vi "Gran result.vi"(6 "first i":u8, 7 "F1":dbl[](array[numeric]) format="%.7f", 8 "length":u8, 9 "Vo":dbl=100.0 format="%.2f", 10 "Nt":dbl=0.05 format="%.2f", 11 "Vt":dbl[](array[numeric]) format="%.5f") -> (0 "graph":cluster{"Vt":dbl[], "F1":dbl[]}[](array[cluster]) {"F1" format="%.2f"; "Vt" format="%.2f"}, 1 "r":dbl=0.5 format="%.6f", 2 "Est. Nt":dbl=0.05 format="%.6f", 3 "ANC":dbl=0.5 format="%.6f", 5 "Ve":dbl=0.5 format="%.6f")   [LabVIEW 2012]
uses:
  <vilib>/Analysis/NI_AALPro.lvlib
  <vilib>/gmath/NI_Gmath.lvlib
panel:
  out "XY Graph":cluster{"Va":dbl[], "F1":dbl[]}[](graph)
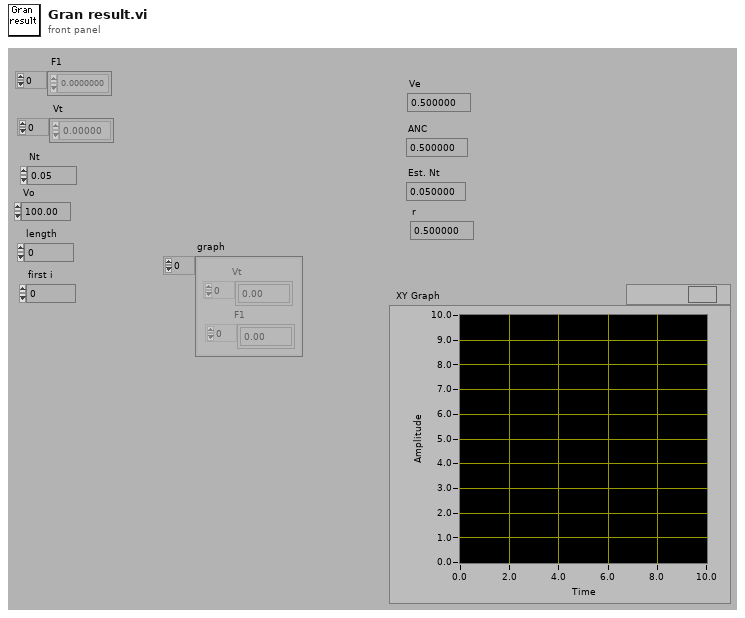
[diagram p1: front panel]
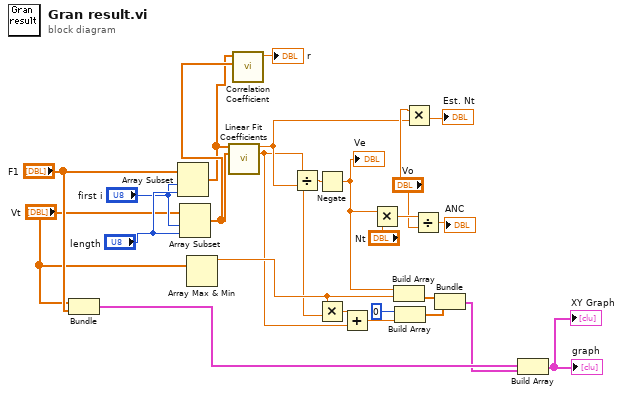
[diagram p0: block diagram]
diagram:
  n1 = Bundle("Vt"="Vt", "F1"="F1") -> (w10:cluster{"Vt":dbl[], "F1":dbl[]})  [unwired: 1 in]
  n2 = Array Subset(array="F1", index="first i", length="length") -> (w2:dbl[])
  n3 = Array Subset(array="Vt", index="first i", length="length") -> (w3:dbl[])
  n4 = Array Max & Min(array="Vt") -> (max value=w11:dbl)  [unwired: 3 out]
  n5 = call <vilib>:"Linear Fit Coefficients.vi"("Y"=w2, "X"=w3) -> ("slope"=w5:dbl, "intercept"=w4:dbl)  [unwired: 11 in, 1 out]
  n6 = call <vilib>:"Correlation Coefficient.vi"("Y"=w3, "X"=w2) -> ("correlation coefficient r"=→"r":dbl)  [unwired: 8 in, 1 out]
  n7 = Divide(x=w4, y=w5) -> (x/y=w22:dbl)
  n8 = Negate(x=w22) -> (-x=w13:dbl)
  "Ve" <- w13
  n9 = Multiply(x=w11, y=w5) -> (x*y=w8:dbl)
  n10 = Add(x=w8, y=w4) -> (x+y=w7:dbl)
  n11 = Multiply(x=w13, y="Nt") -> (x*y=w25:dbl)
  n12 = Build Array(w13, w11) -> (w23:dbl[])
  n13 = Build Array(0, w7) -> (w15:dbl[])
  n14 = Multiply(x="Vo", y=w5) -> (x*y=→"Est. Nt":dbl)
  n15 = Divide(x=w25, y="Vo") -> (x/y=→"ANC":dbl)
  n16 = Bundle(w23, w15) -> (w9:cluster{dbl[], dbl[]})  [unwired: 1 in]
  n17 = Build Array(w10, w9) -> (→"graph" →"XY Graph":cluster{"Vt":dbl[], "F1":dbl[]}[])
